vi "Main_10b.vi"() -> ()   [LabVIEW 2020]
panel:
  out "Array":bool[][](array[boolean])
  out "X":i32
  out "Value":i32[](array[numeric])
  in  "Example 2":string="addx 15\naddx -11\naddx 6\naddx -3\naddx 5\naddx -1\naddx -8\naddx 13\naddx 4\nnoop\naddx -1\naddx 5\naddx -1\naddx 5\naddx -1\naddx 5\naddx -1\naddx 5\naddx -1\naddx -35\naddx 1\naddx 24\naddx -19\naddx 1\naddx 16\naddx -11\nnoop\nnoop\naddx 21\naddx -15\nnoop\nnoop\naddx -3\naddx 9\naddx 1\naddx -3\naddx 8\naddx 1\naddx 5\nnoop\nnoop\nnoop\nnoop\nnoop\naddx -36\nnoop\naddx 1\naddx 7\nnoop\nnoop\nnoop\naddx 2\naddx 6\nnoop\nnoop\nnoop\nnoop\nnoop\naddx 1\nnoop\nnoop\naddx 7\naddx 1\nnoop\naddx -13\naddx 13\naddx 7\nnoop\naddx 1\naddx -33\nnoop\nnoop\nnoop\naddx 2\nnoop\nnoop\nnoop\naddx 8\nnoop\naddx -1\naddx 2\naddx 1\nnoop\naddx 17\naddx -9\naddx 1\naddx 1\naddx -3\naddx 11\nnoop\nnoop\naddx 1\nnoop\naddx 1\nnoop\nnoop\naddx -13\naddx -19\naddx 1\naddx 3\naddx 26\naddx -30\naddx 12\naddx -1\naddx 3\naddx 1\nnoop\nnoop\nnoop\naddx -9\naddx 18\naddx 1\naddx 2\nnoop\nnoop\naddx 9\nnoop\nnoop\nnoop\naddx -1\naddx 2\naddx -37\naddx 1\naddx 3\nnoop\naddx 15\naddx -21\naddx 22\naddx -6\naddx 1\nnoop\naddx 2\naddx 1\nnoop\naddx -10\nnoop\nnoop\naddx 20\naddx 1\naddx 2\naddx 2\naddx -6\naddx -11\nnoop\nnoop\nnoop"
  out "sum":i32
  in  "Puzzle":string="addx 1\naddx 5\nnoop\naddx -1\nnoop\naddx 3\naddx 29\naddx -1\naddx -21\naddx 5\nnoop\naddx -20\naddx 21\naddx 2\naddx 8\naddx -1\nnoop\nnoop\nnoop\nnoop\naddx 6\naddx -1\naddx -37\naddx 40\naddx -10\naddx -25\naddx 5\naddx 2\naddx 5\nnoop\nnoop\nnoop\naddx 21\naddx -20\naddx 2\nnoop\naddx 3\naddx 2\naddx -5\naddx 12\naddx 3\nnoop\naddx 2\naddx 3\naddx -2\naddx -37\naddx 1\naddx 5\naddx 3\naddx -2\naddx 2\naddx 29\naddx -22\naddx 13\nnoop\naddx -8\naddx -6\naddx 7\naddx 2\nnoop\naddx 7\naddx -2\naddx 5\naddx 2\naddx -26\naddx -11\nnoop\nnoop\naddx 6\naddx 1\naddx 1\nnoop\naddx 4\naddx 5\nnoop\nnoop\naddx -2\naddx 3\nnoop\naddx 2\naddx 5\naddx 2\naddx -22\naddx 27\naddx -1\naddx 1\naddx 5\naddx 2\nnoop\naddx -39\naddx 22\nnoop\naddx -15\naddx 3\naddx -2\naddx 2\naddx -2\naddx 9\naddx 3\nnoop\naddx 2\naddx 3\naddx -2\naddx 2\nnoop\nnoop\nnoop\naddx 5\naddx -17\naddx 24\naddx -7\naddx 8\naddx -36\naddx 2\naddx 3\naddx 33\naddx -32\naddx 4\naddx 1\nnoop\naddx 5\nnoop\nnoop\naddx 20\naddx -15\naddx 4\nnoop\naddx 1\nnoop\naddx 4\naddx 6\naddx -30\naddx 30\nnoop\nnoop\nnoop\nnoop\nnoop"
  in  "Example":string="noop\naddx 3\naddx -5"
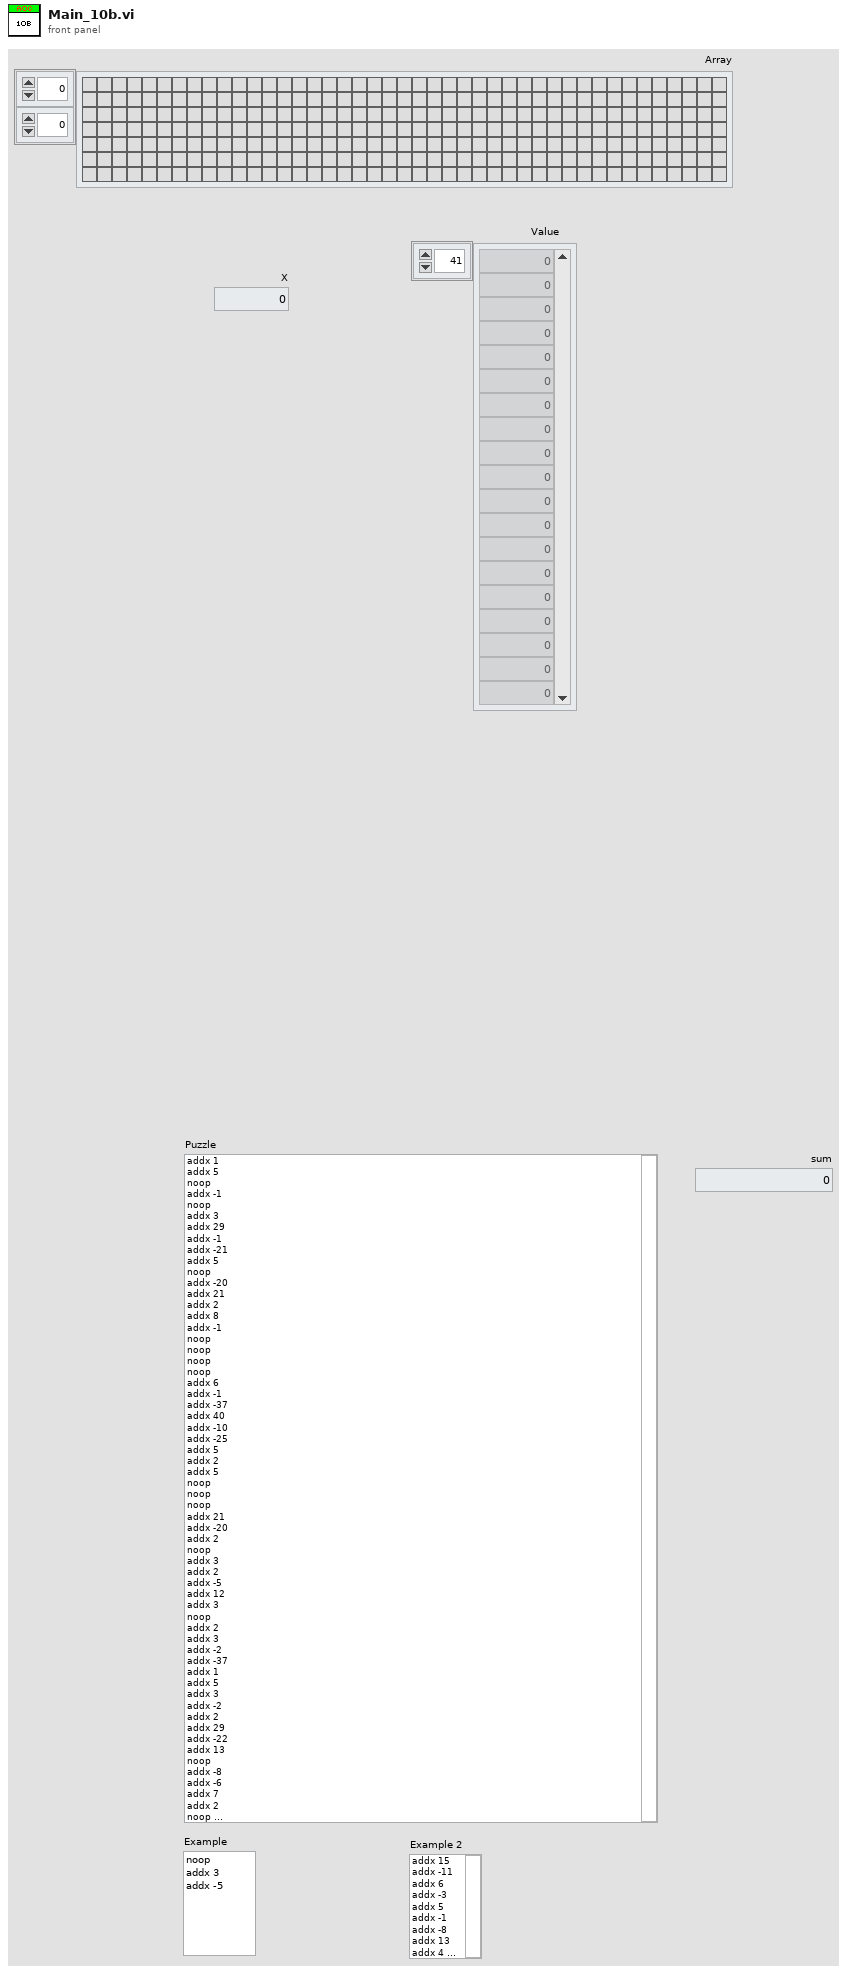
[diagram p1: front panel]
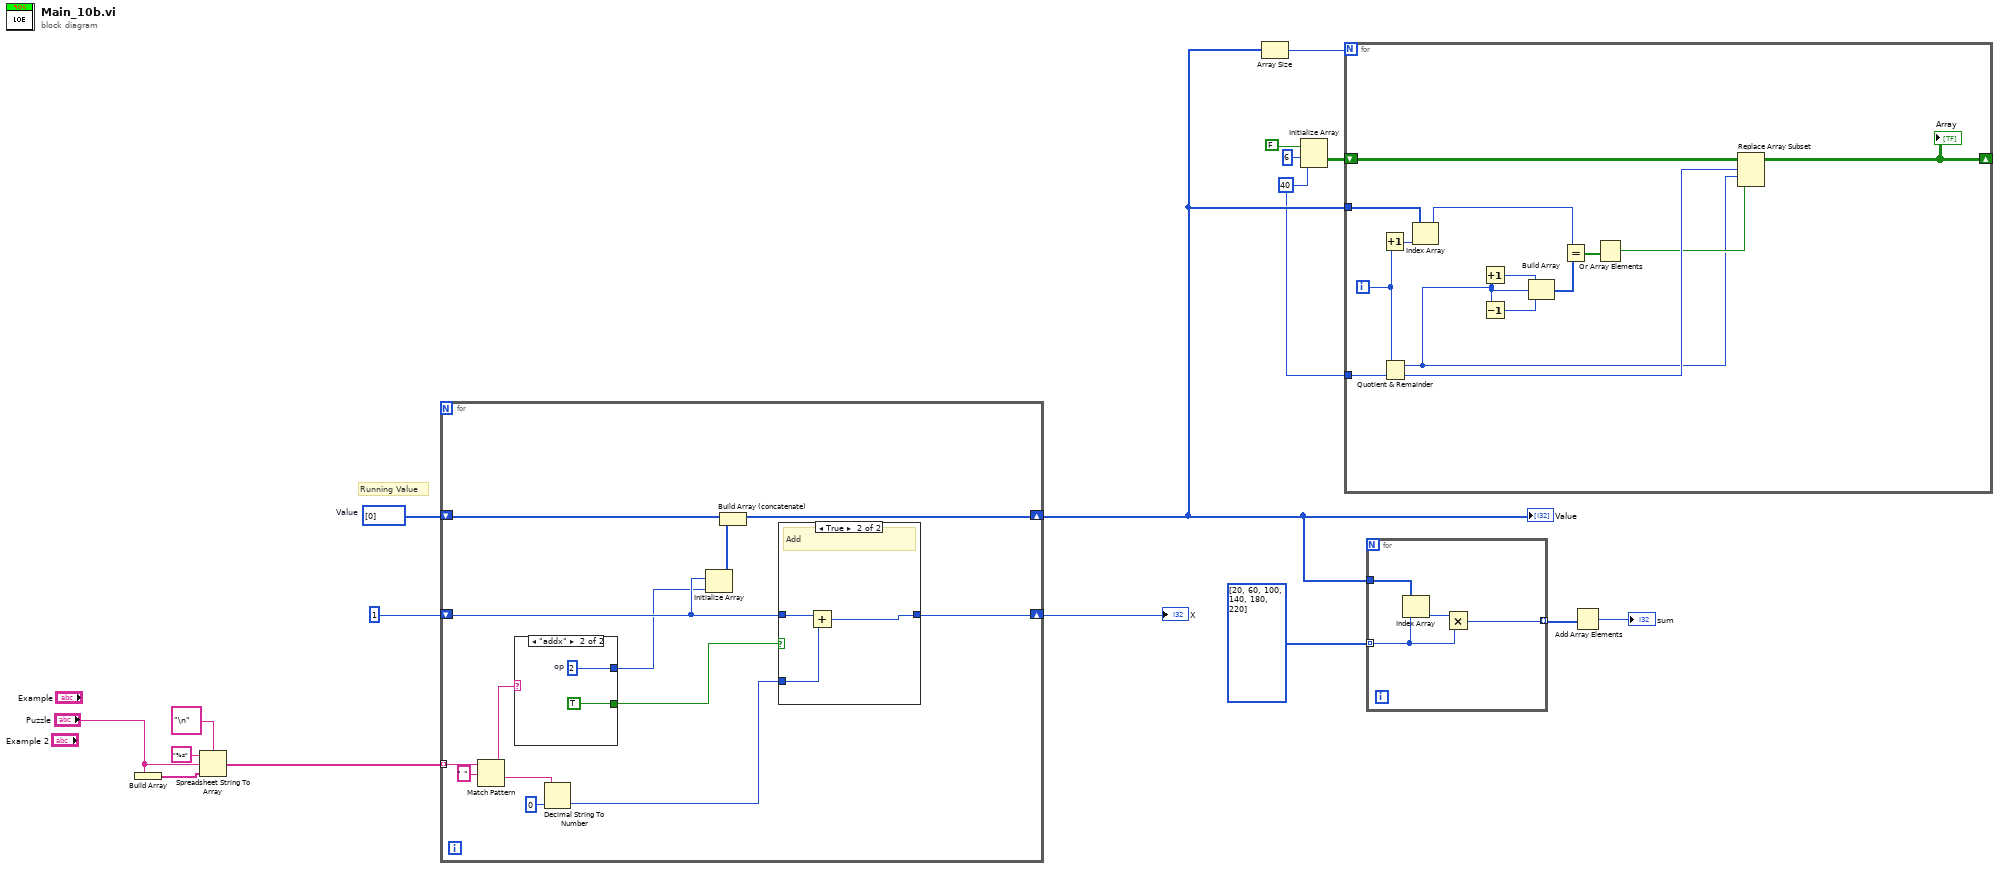
[diagram p0: block diagram]
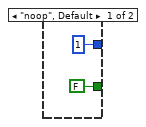
[diagram p2: hidden frame]
diagram:
  w2 = 40 ("dimension size")
  w14 = i32[] [0]  # Value
  # "Running Value"
  n1 = Build Array("Puzzle") -> (w12:string[])
  n2 = Spreadsheet String To Array(delimiter (Tab)="\n", format string="%s", spreadsheet string="Puzzle", array type (2D Dbl)=w12) -> (array=w13:string[])
  n3 = for {
    shift-right: [w26] -> w11
    shift-left: 1 -> [w28]
    shift-right: [w27] -> w4
    shift-left: w14 -> [w30]
    tunnel: w13 -> [w25] mode=indexing
    n4 = Match Pattern(string=w25, regular expression=" ") -> (before substring=w20:string, after substring=w24:string)  [unwired: 1 in, 2 out]
    n5 = case shown="\"addx\"" w20 {
      tunnel: [1 ("op") w34] -> w19
      tunnel: [FALSE TRUE] -> w18
      frame "noop", Default {
      }
      frame "addx" {
        w34 = 2  # op
      }
    }
    n6 = Decimal String To Number(string=w24, default (0L)=0 ("default (0 I32)")) -> (number=w21:i32)  [unwired: 1 in, 1 out]
    n7 = Initialize Array(w28, w19) -> (w29:i32[])
    n8 = Build Array (concatenate)(w30, w29) -> (w27:i32[])
    n9 = case shown="True" w18 {
      tunnel: w28 -> [w35 w38]
      tunnel: w21 -> [_ w37]
      tunnel: [w35 w36] -> w26
      frame False {
        # "noop"
      }
      frame True {
        # "Add"
        n10 = Add(x=w38, y=w37) -> (x+y=w36:i32)
      }
    }
  }
  "Value" <- w4
  "X" <- w11
  n11 = Array Size(array=w4) -> (size(s)=w3:i32)
  n12 = Initialize Array(FALSE ("Boolean"), 6 ("dimension size"), w2) -> (w5:bool[][])
  n13 = for {
    N: w3 -> [_]
    tunnel: w4 -> [w42]
    shift-right: [w51] -> _
    shift-left: w5 -> [w52]
    tunnel: w2 -> [w41]
    i -> [w40]
    n14 = Increment(x=w40) -> (x+1=w44:i32)
    n15 = Quotient & Remainder(x=w40, y=w41) -> (x-y*floor(x/y)=w39:i32, floor(x/y)=w46:i32)
    n16 = Index Array(array=w42, index=w44) -> (element=w43:i32)
    n17 = Increment(x=w39) -> (x+1=w50:i32)
    n18 = Decrement(x=w39) -> (x-1=w49:i32)
    n19 = Build Array(w50, w39, w49) -> (w48:i32[])
    n20 = Equal?(x=w43, y=w48) -> (x = y?=w47:bool[])
    n21 = Or Array Elements(Boolean array=w47) -> (logical OR=w45:bool)
    n22 = Replace Array Subset(array=w52, new element=w45, index (row)=w46, index (col)=w39) -> (w51:bool[][])
    "Array" <- w51
  }
  n23 = for {
    tunnel: i32[] [20, 60, 100, 140, 180, 220] ("Value") -> [w54] mode=indexing
    tunnel: w4 -> [w56]
    tunnel: [w53] -> w9 mode=indexing
    n24 = Index Array(array=w56, index=w54) -> (element=w55:i32)
    n25 = Multiply(x=w55, y=w54) -> (x*y=w53:i32)
  }
  n26 = Add Array Elements(numeric array=w9) -> (sum=→"sum":i32)
